vi "PS1-_PS2+_Connection.vi"(0 "On/Off":bool, 1 "Delay Time (s)":dbl=1.0, 3 "error in":errorcluster) -> (10 "error out":errorcluster)   [LabVIEW 2015]
panel:
  # "port2/line1"
  # "ON means close relay\nOFF means open relay"
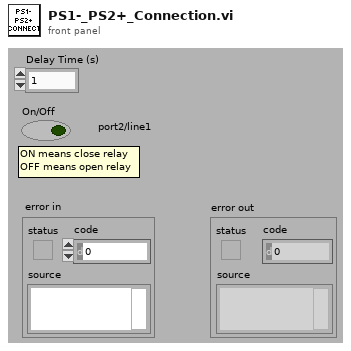
[diagram p1: front panel]
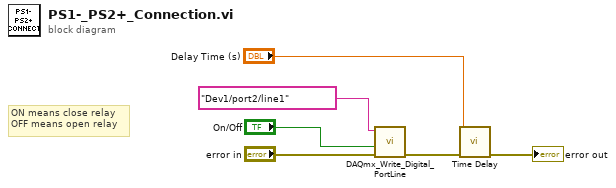
[diagram p0: block diagram]
diagram:
  # "ON means close relay\nOFF means open relay"
  n1 = call "DAQmx_Write_Digital_PortLine.vi"("Device/Ports/Lines"="Dev1/port2/line1", "Boolean"="On/Off", "error in"="error in") -> ("error out"=w4:errorcluster)  [unwired: 6 in, 1 out]
  n2 = call "Time Delay"("error in (no error)"=w4, "Delay Time (s)"="Delay Time (s)") -> ("error out"=→"error out":errorcluster)  [unwired: 9 in]
